vi "Dynamic_call_global.ph.vi"() -> ()   [LabVIEW 2017]
panel:
  in  "Desired NorthWest Window Open %":dbl
  in  "Desired East Window Open %":dbl
  in  "Desired SouthWest Window Open %":dbl
  in  "Pre_Analysis_Plugin":string
  in  "Take LDA PWA & An":refnum<vi>
  in  "Initial Plug Ins Extra":string[](array[string])
  in  "Per Block Plug Ins Extra":string[](array[string])
  in  "GPIB_Server.vi":refnum<vi>
  out "EnFlo Hub running?":bool
  in  "Final Plug Ins":string[](array[string])
  in  "Per Block Plug Ins":string[](array[string])
  in  "Initial Plug Ins":string[](array[string])
  in  "Error Cluster":errorcluster
  in  "Client Name":string
  in  "Scanning Valve Driver":refnum<vi>
  in  "Program Active server":refnum<vi>
  in  "Opened VIs":string[](array[string])
  in  "Plug in":refnum<vi>
  in  "Analogue Input":refnum<vi>
  in  "Plug in values":string[](array[string])
  in  "Plug in titles":string[](array[string])
  in  "Remote Subvi Opened":refnum<k4>
  in  "VI name to launch":string
  in  "Call Remote Subvi":refnum<k4>
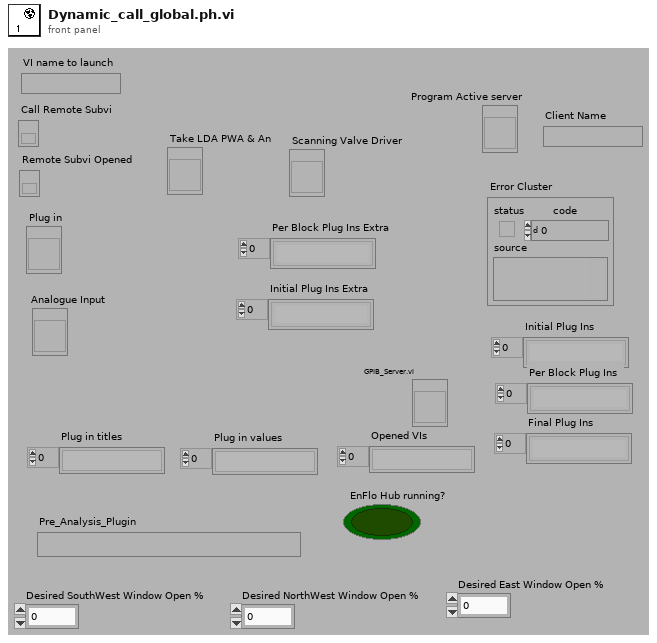
[diagram p1: front panel]
diagram:
